vi "CRYOpen Step by Legend.vi"(9 "Active Row":i32, 10 "MCListbox Ref In":refnum<vi>, 11 "Type":enum16{"Curves", "Values", "Results", "WFM"}(ring)) -> ()   [LabVIEW 2013]
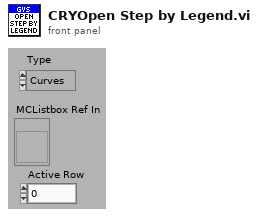
[diagram p1: front panel]
types:
  T1 = typedef "CRYWaveform Cluster Array.ctl" = T2[]
  T2 = typedef "CRYWaveform Cluster.ctl" = cluster{"Waveform":cluster{"X0":dbl, "dX":dbl, "Y":sgl[]}, "X data":u16, "Y data":u16, "Y axis":u16, "X unit":string, "Y unit":string, "Y dB ref":dbl, "display Y":bool, "display X":bool, "Overload?":bool, "Test Info":string, "Step No.":i32, "Name":string, "protected":bool, "Sqc history":string[], "Signal Channel ID":i32, "Plot Settings":cluster{"Color":u32, "Interpolation":u8, "Point Style":u8, "Line Style":u8, "Point Color":u32, "Line Width":u8, "Bar Plot Style":u8, "Fill To":i16}, "AutoProtect":bool}
  T3 = typedef "CRYResult Cluster Array.ctl" = T4[]
  T4 = typedef "CRYResult Cluster.ctl" = cluster{"Name":string, "Margin":dbl, "unit":string, "Verdict":bool, "Limit":string, "Max/Min":string, "protected":bool, "Step No.":i32, "Test Info":string, "AutoProtect":bool}
  T5 = typedef "CRYData Cluster Array.ctl" = T6[]
  T6 = typedef "CRYData Cluster.ctl" = cluster{"Name":string, "Curve":cluster{"x":dbl, "y":dbl, "z":dbl}[], "X data":u16, "Y data":u16, "Z data":u16, "X axis":u16, "Y axis":u16, "Z axis":u16, "X unit":string, "Y unit":string, "Z unit":string, "X dB ref":dbl, "Y dB ref":dbl, "Z dB ref":dbl, "single val":bool, "protected":bool, "display X":bool, "display Y":bool, "display Z":bool, "Test Info":string, "Step No.":i32, "Plot Settings":cluster{"Color":u32, "Interpolation":u8, "Point Style":u8, "Line Style":u8, "Point Color":u32, "Line Width":u8, "Bar Plot Style":u8, "Fill To":i16}, "AutoProtect":bool}
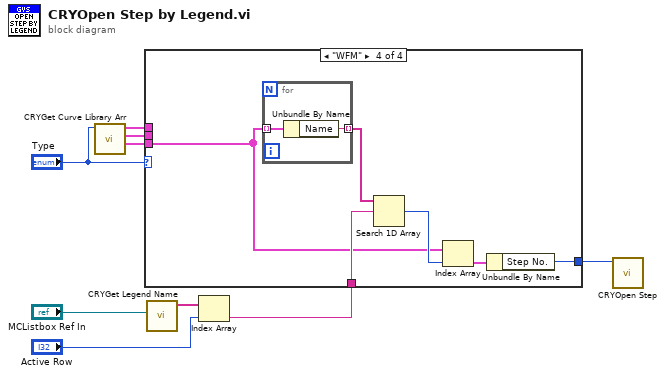
[diagram p0: block diagram]
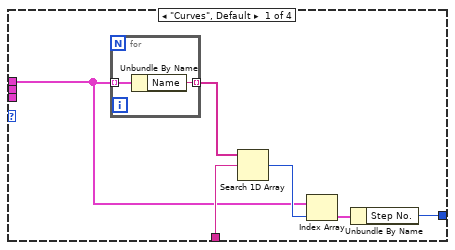
[diagram p2: hidden frame]
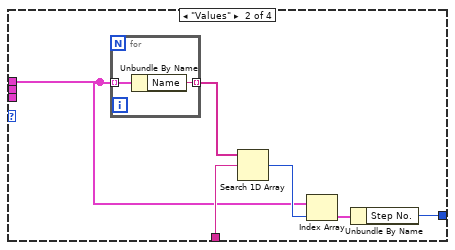
[diagram p3: hidden frame]
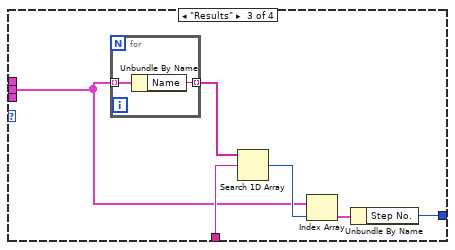
[diagram p4: hidden frame]
diagram:
  n1 = call "CRYGet Curve Library Arr.vi"("Type In"="Type") -> ("Waveforms"=w1:T1, "Results"=w2:T3, "Curves/Values"=w3:T5)  [unwired: 8 in]
  n2 = call "CRYGet Legend Name.vi"("MCListbox Refnum"="MCListbox Ref In") -> ("Names Out"=w9:string[])  [unwired: 1 in, 9 out]
  n3 = Index Array(array=w9, index="Active Row") -> (element=w8:string)
  n4 = case shown="\"WFM\"" "Type" {
    tunnel: w8 -> [w14 w22 w30 w38]
    tunnel: [w11 w19 w27 w35] -> w5
    tunnel: w3 -> [w10 w18 _ _]
    tunnel: w2 -> [_ _ w26 _]
    tunnel: w1 -> [_ _ _ w34]
    frame "Curves", Default {
      n5 = for {
        tunnel: w10 -> [w17] mode=indexing
        tunnel: [w16] -> w15 mode=indexing
        n6 = Unbundle By Name(w17) -> ("Name"=w16:string)
      }
      n7 = Search 1D Array(1D array=w15, element=w14) -> (index of element=w13:i32)  [unwired: 1 out]
      n8 = Index Array(array=w10, index=w13) -> (element=w12:T6)
      n9 = Unbundle By Name(w12) -> ("Step No."=w11:i32)
    }
    frame "Values" {
      n10 = for {
        tunnel: w18 -> [w25] mode=indexing
        tunnel: [w24] -> w23 mode=indexing
        n11 = Unbundle By Name(w25) -> ("Name"=w24:string)
      }
      n12 = Search 1D Array(1D array=w23, element=w22) -> (index of element=w21:i32)  [unwired: 1 out]
      n13 = Index Array(array=w18, index=w21) -> (element=w20:T6)
      n14 = Unbundle By Name(w20) -> ("Step No."=w19:i32)
    }
    frame "Results" {
      n15 = for {
        tunnel: w26 -> [w33] mode=indexing
        tunnel: [w32] -> w31 mode=indexing
        n16 = Unbundle By Name(w33) -> ("Name"=w32:string)
      }
      n17 = Search 1D Array(1D array=w31, element=w30) -> (index of element=w29:i32)  [unwired: 1 out]
      n18 = Index Array(array=w26, index=w29) -> (element=w28:T4)
      n19 = Unbundle By Name(w28) -> ("Step No."=w27:i32)
    }
    frame "WFM" {
      n20 = for {
        tunnel: w34 -> [w41] mode=indexing
        tunnel: [w40] -> w39 mode=indexing
        n21 = Unbundle By Name(w41) -> ("Name"=w40:string)
      }
      n22 = Search 1D Array(1D array=w39, element=w38) -> (index of element=w37:i32)  [unwired: 1 out]
      n23 = Index Array(array=w34, index=w37) -> (element=w36:T2)
      n24 = Unbundle By Name(w36) -> ("Step No."=w35:i32)
    }
  }
  n25 = call "CRYOpen Step.vi"("Step No."=w5) -> ()  [unwired: 11 out]
